vi "Create Public Test Methods.vi"(8 "error in (no error)":errorcluster, 11 "Test Double Factory in":refnum<class "Test Double Factory.lvclass">) -> (0 "error out":errorcluster, 3 "Test Double Factory out":refnum<class "Test Double Factory.lvclass">)   [LabVIEW 2020, in "Test Double Factory.lvclass"]
uses:
  Test Double Factory.lvclass
  Test Double Factory.lvclass/Test Double Factory.ctl
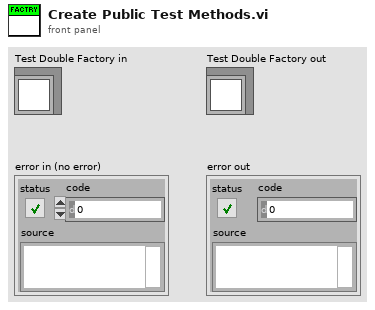
[diagram p1: front panel]
types:
  T1 = enum32{"invalid scope", "public", "private", "protected", "community"}
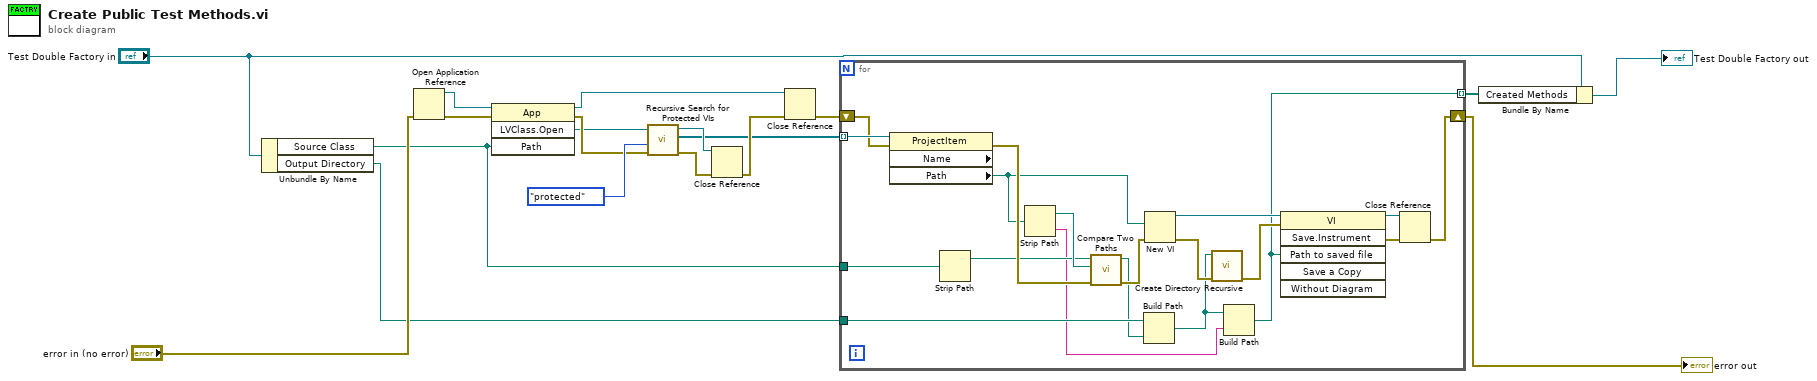
[diagram p0: block diagram]
diagram:
  n1 = Unbundle By Name("Test Double Factory in") -> ("Source Class"=w6:path, "Output Directory"=w9:path)
  n2 = Open Application Reference(8:"error in (no error)") -> (0:w3:errorcluster, 3:w17:refnum<vi>)  [unwired: 3 in]
  n3 = invoke class="App" method="LVClass.Open"(reference=w17, error in=w3, "Path"=w6) -> (reference out=w7:refnum<vi>, error out=w2:errorcluster, "LVClass.Open"=w1:refnum<vi>)  [unwired: 1 in, 1 out]
  n4 = call "Recursive Search for Protected VIs.vi"("error in (no error)"=w2, "Scope"=T1."protected", "LVClassLibrary in"=w1) -> ("error out"=w14:errorcluster, "Protected VI Refs"=w4:refnum<vi>[], "LVClassLibrary out"=w13:refnum<vi>)  [unwired: 6 in]
  n5 = Close Reference(reference=w13, error in (no error)=w14) -> (error out=w15:errorcluster)
  n6 = Close Reference(reference=w7, error in (no error)=w15) -> (error out=w8:errorcluster)
  n7 = for {
    tunnel: w4 -> [w37] mode=indexing
    shift-right: [w32] -> w10
    shift-left: w8 -> [w33]
    tunnel: w6 -> [w31]
    tunnel: w9 -> [w27]
    tunnel: [w19] -> w11 mode=indexing
    n8 = property class="ProjectItem" props=["Name", "Path"](reference=w37, error in=w33) -> (error out=w30:errorcluster, "Path"=w28:path)  [unwired: 2 out]
    n9 = Strip Path(path=w31) -> (stripped path=w22:path)  [unwired: 1 out]
    n10 = Strip Path(path=w28) -> (stripped path=w23:path, name=w20:string)
    n11 = call <vilib>:"Compare Two Paths.vi"("error in (no error)"=w30, "Path 2"=w23, "Path 1"=w22) -> ("error out"=w29:errorcluster, "Relative Path from 1 to 2"=w26:path)  [unwired: 5 in, 2 out]
    n12 = Build Path(base path=w27, name or relative path=w26) -> (appended path=w21:path)
    n13 = New VI(8:w29, 10:w28) -> (0:w25:errorcluster, 3:w36:refnum<vi>)  [unwired: 5 in]
    n14 = call <vilib>:"Create Directory Recursive.vi"("error in (no error)"=w25, "directory"=w21) -> ("error out"=w24:errorcluster)  [unwired: 3 in, 2 out]
    n15 = Build Path(base path=w21, name or relative path=w20) -> (appended path=w19:path)
    n16 = invoke class="VI" method="Save.Instrument"(reference=w36, error in=w24, "Path to saved file"=w19) -> (reference out=w34:refnum<vi>, error out=w35:errorcluster)  [unwired: 3 in, 4 out]
    n17 = Close Reference(reference=w34, error in (no error)=w35) -> (error out=w32:errorcluster)
  }
  "error out" <- w10
  n18 = Bundle By Name(cluster="Test Double Factory in", "Created Methods"=w11) -> (→"Test Double Factory out":refnum<class "Test Double Factory.lvclass">)
